vi "buttonFGV.vi"(10 "command":T1, 11 "Boolean in":refnum<vi>) -> (0 "Path":path, 1 "select subPanel":bool, 3 "Boolean out":refnum<vi>)   [LabVIEW 2020]
uses:
  Controls/controlFGV_TYPDEF.ctl
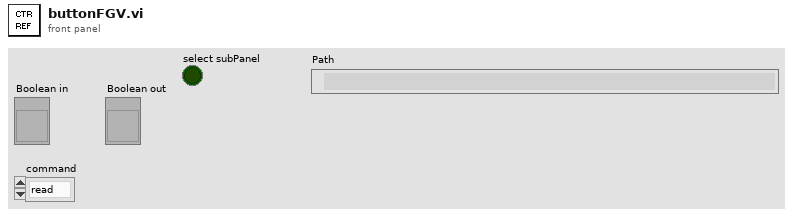
[diagram p1: front panel]
types:
  T1 = typedef "controlFGV_TYPDEF.ctl" = enum16{"read", "write", "clear"}
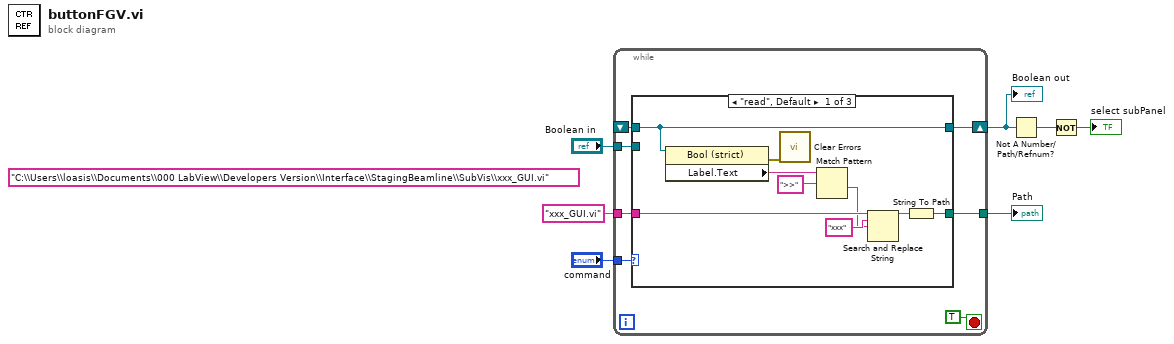
[diagram p0: block diagram]
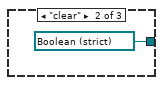
[diagram p2: hidden frame]
diagram:
  (unwired) "C:\\Users\\loasis\\Documents\\000 LabView\\Developers Version\\Interface\\StagingBeamline\\SubVis\\xxx_GUI.vi" ("vi path")
  n1 = while {
    tunnel: "command" -> [w14]
    shift-right: [w10] -> w3
    shift-left: _ -> [w12]
    tunnel: "Boolean in" -> [w13]
    tunnel: "xxx_GUI.vi" ("vi path") -> [w9]
    tunnel: [w8] -> w1
    stop <- TRUE stop-if-true
    n2 = case shown="\"read\", Default" w14 {
      tunnel: w13 -> [_ _ w25]
      tunnel: [w23 refnum<vi> refnum ("Boolean in") w25] -> w10
      tunnel: w12 -> [w23 _ _]
      tunnel: w9 -> [w20 _ _]
      tunnel: [w16 _ _] -> w8
      frame "read", Default {
        n3 = property class="Bool (strict)"(reference=w23) -> (error out=w15:errorcluster, "Label.Text"=w22:string)  [unwired: 1 in, 1 out]
        n4 = call <vilib>:"Clear Errors.vi"("error in (no error)"=w15) -> ()  [unwired: 5 in, 2 out]
        n5 = Match Pattern(string=w22, regular expression=">>") -> (after substring=w18:string)  [unwired: 1 in, 3 out]
        n6 = Search and Replace String(input string=w20, search string="xxx", replace string=w18) -> (result string=w17:string)  [unwired: 5 in, 3 out]
        n7 = String To Path(string=w17) -> (path=w16:path)
      }
      frame "clear" {
      }
      frame "write" {
      }
    }
  }
  "Boolean out" <- w3
  "Path" <- w1
  n8 = Not A Number/Path/Refnum?(number/path/refnum=w3) -> (NaN/Path/Refnum?=w5:bool)
  n9 = Not(x=w5) -> (.not. x?=→"select subPanel":bool)
